vi "stop.vi"(8 "error in (no error)":errorcluster, 11 "HSDIO in":refnum<class "HSDIO.lvclass">) -> (0 "error out":errorcluster, 3 "HSDIO out":refnum<class "HSDIO.lvclass">)   [LabVIEW 2013, in "HSDIO.lvclass"]
uses:
  HSDIO.lvclass
  HSDIO.lvclass/HSDIO.ctl
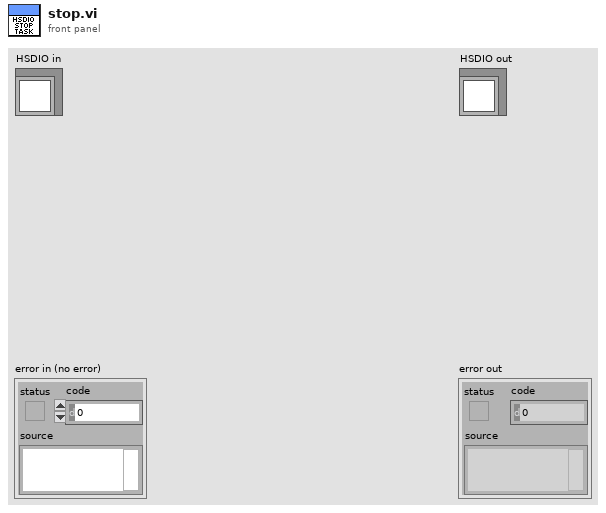
[diagram p1: front panel]
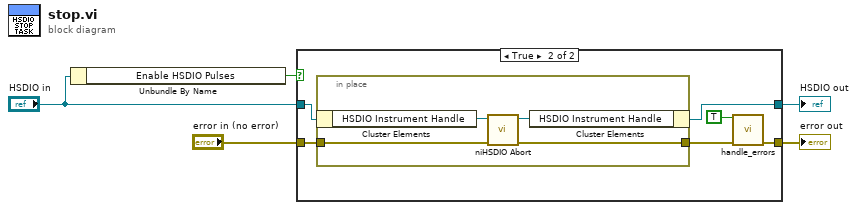
[diagram p0: block diagram]
diagram:
  n1 = Unbundle By Name("HSDIO in") -> ("Enable HSDIO Pulses"=w3:bool)
  n2 = case shown="True" w3 {
    tunnel: [w7 w11] -> w4
    tunnel: "error in (no error)" -> [w7 w13]
    tunnel: "HSDIO in" -> [w6 w9]
    tunnel: [w6 w8] -> w1
    frame False {
    }
    frame True {
      n3 = in-place {
        in-place-border: w13 -> [w17]
        in-place-border: [w16] -> w12
        n4 = in-place-cluster #1(w9) -> ("HSDIO Instrument Handle"=w15:refnum<k15>)
        n5 = call <instrlib>:"niHSDIO Abort.vi"("error in (no error)"=w17, "instrument handle"=w15) -> ("error out"=w16:errorcluster, "instrument handle out"=w14:refnum<k15>)  [unwired: 8 in]
        n6 = in-place-cluster #1("HSDIO Instrument Handle"=w14) -> (w8:refnum<class "HSDIO.lvclass">)
      }
      n7 = call "handle_errors.vi"("Exit Operation"=TRUE ("Exit Measurement"), "error in (no error)"=w12) -> ("error out"=w11:errorcluster)  [unwired: 13 in]
    }
  }
  "error out" <- w4
  "HSDIO out" <- w1
